vi "Waveform_Generation_SubVI.vi"(8 "ADSR in":dbl[](array[numeric]), 11 "Main Data Cluster in":T1={"Notes Frequency Array"=[], "Main Waveform Type"=enum."Sine", "Waveform"={"t0"=timestamp(0 s since 1904-01-01), "dt"=1.0, "Y"=[]}, "Main Current Note"=0, "Octave Range Offset"=0, "sound format"={"sample rate (S/s)"=22050.0, "number of channels"=2, "bits per sample"=16}, "Task ID"=0, "Note Duration"=0.0, "Volume"=0.0, "ADSR Envelope Cluster"={"Decay"=0, "Sustain"=0, "Attack"=0, "Release"=0}, "Playing?"=FALSE, "Pitch LFO"={"Rate"=0.0, "Ammount"=0.0}, "device ID"=0, "Filter Section"={"Lowpass Freq"=0.0, "Highpass Freq"=0.0, "Enable"=FALSE}, "Distortion"={"Distortion level"=0.0, "Enable"=FALSE}, "Secondary Waveform Type"=enum."Sine", "Secondary Frequency"=0.0, "Secondary Blend"=0.0, "Envelope XY Graph"={[], []}, "Buffer Number"=0, "End of Sequence?"=FALSE} {"task ID" format="%.0x"}) -> (2 "Signal Array out":dbl[](array[numeric]), 3 "dt out":dbl)   [LabVIEW 2019]
doc: "This SubVI generates a specified waveform.\n\nIN: Note Duration in; Sample Rate in; Note Freq in; Waveform Type in; Envelope Array in;\nOUT: dt out; Signal Array out;"
uses:
  <vilib>/Analysis/NI_AALBase.lvlib
  <vilib>/numeric/Random Number (Range) DBL.vi
  controls/#typedef_Waveform_Type.ctl
  <vilib>/sound2/lvsound2.llb/Sound Data Format.ctl
  <vilib>/sound2/lvsound2.llb/Sound Output Task ID.ctl
  controls/#typedef_Data_Cluster.ctl
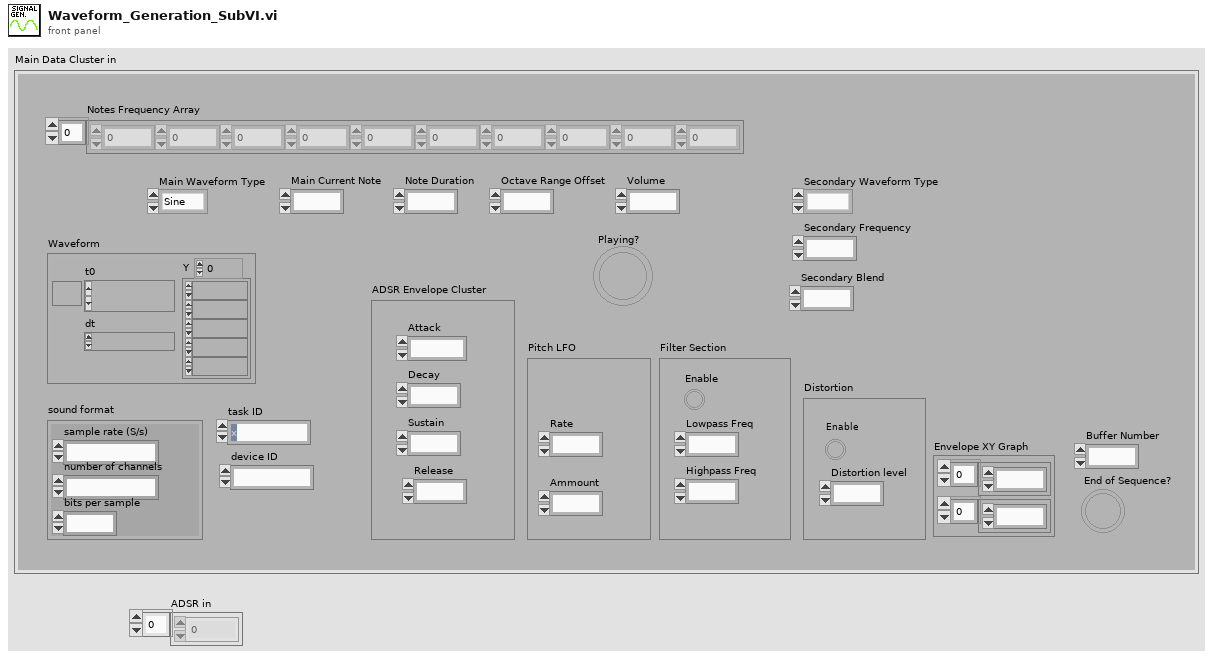
[diagram p1: front panel]
types:
  T1 = typedef "#typedef_Data_Cluster.ctl" = cluster{"Notes Frequency Array":dbl[], "Main Waveform Type":T2, "Waveform":waveform(dbl), "Main Current Note":i32, "Octave Range Offset":u32, "sound format":T3, "Task ID":T4, "Note Duration":dbl, "Volume":dbl, "ADSR Envelope Cluster":cluster{"Decay":i32, "Sustain":i32, "Attack":i32, "Release":i32}, "Playing?":bool, "Pitch LFO":cluster{"Rate":dbl, "Ammount":dbl}, "device ID":u32, "Filter Section":cluster{"Lowpass Freq":dbl, "Highpass Freq":dbl, "Enable":bool}, "Distortion":cluster{"Distortion level":dbl, "Enable":bool}, "Secondary Waveform Type":T2, "Secondary Frequency":dbl, "Secondary Blend":dbl, "Envelope XY Graph":cluster{dbl[], dbl[]}, "Buffer Number":i32, "End of Sequence?":bool}
  T2 = typedef "#typedef_Waveform_Type.ctl" = enum16{"Sine", "Saw", "Square", "Triangle", "Noise"}
  T3 = typedef "Sound Data Format.ctl" = cluster{"sample rate (S/s)":dbl, "number of channels":i32, "bits per sample":i32}
  T4 = typedef "Sound Output Task ID.ctl" = u32
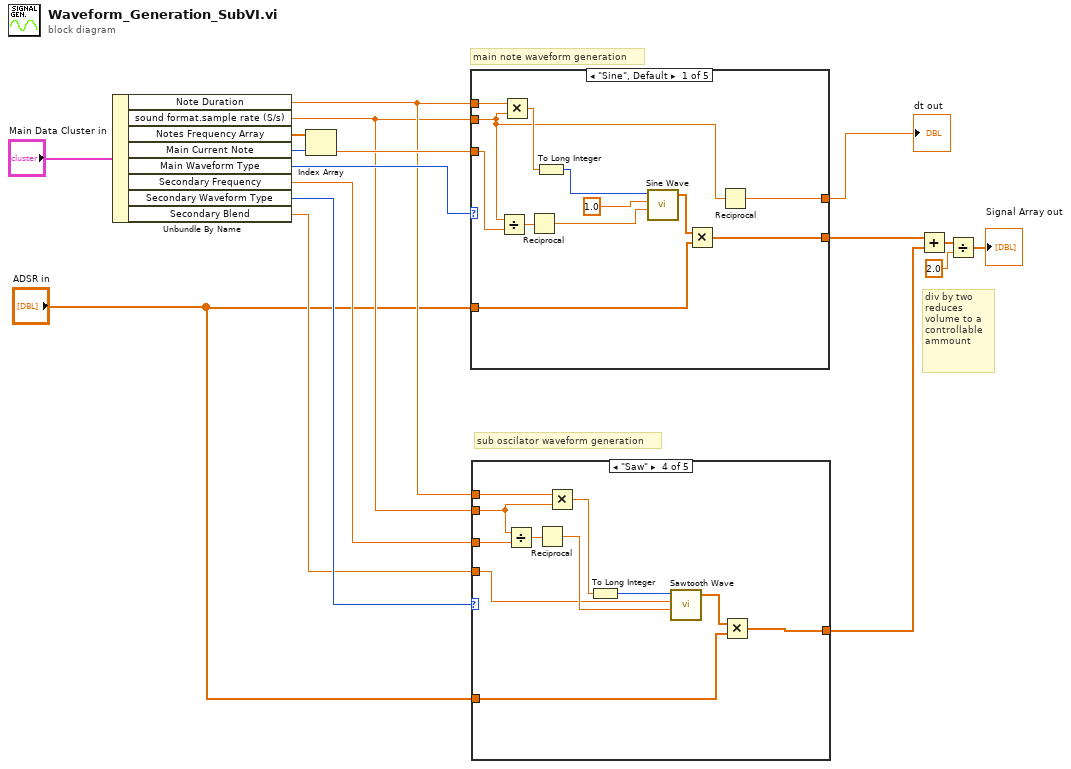
[diagram p0: block diagram]
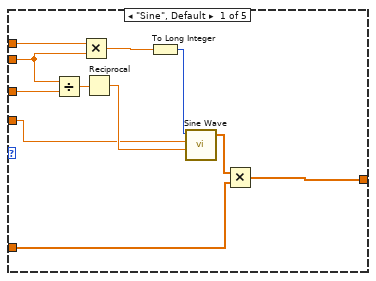
[diagram p2: hidden frame]
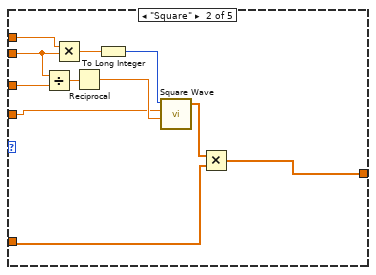
[diagram p3: hidden frame]
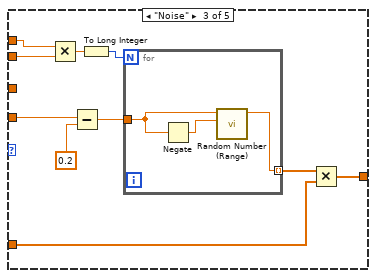
[diagram p4: hidden frame]
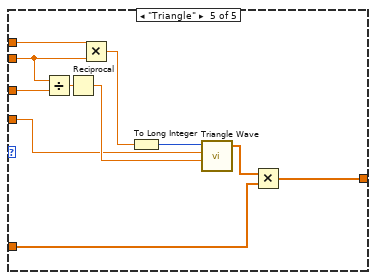
[diagram p5: hidden frame]
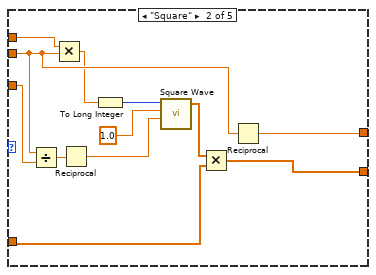
[diagram p6: hidden frame]
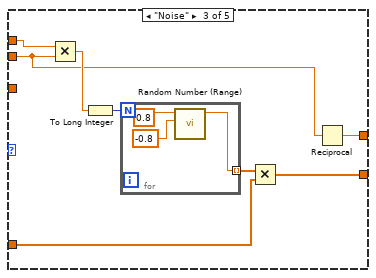
[diagram p7: hidden frame]
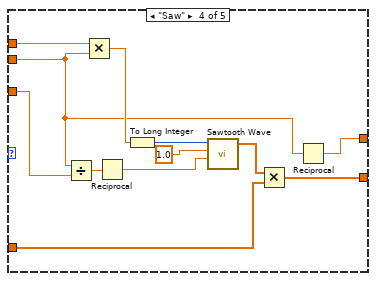
[diagram p8: hidden frame]
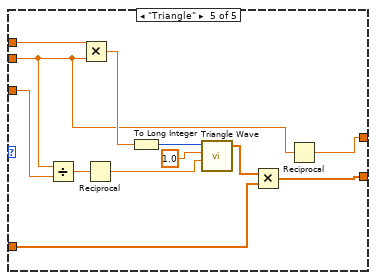
[diagram p9: hidden frame]
diagram:
  # "div by two reduces volume to a controllable ammount"
  # "main note waveform generation"
  # "sub oscilator waveform generation"
  n1 = Unbundle By Name("Main Data Cluster in") -> ("Note Duration"=w11:dbl, "sound format.sample rate (S/s)"=w10:dbl, "Notes Frequency Array"=w15:dbl[], "Main Current Note"=w16:i32, "Main Waveform Type"=w13:T2, "Secondary Frequency"=w9:dbl, "Secondary Waveform Type"=w8:T2, "Secondary Blend"=w7:dbl)
  n2 = Index Array(array=w15, index=w16) -> (element=w14:dbl)
  n3 = case shown="\"Sine\", Default" w13 {
    tunnel: w14 -> [w28 w40 _ w61 w71]
    tunnel: w10 -> [w24 w37 w44 w55 w67]
    tunnel: w11 -> [w27 w39 w48 w62 w74]
    tunnel: "ADSR in" -> [w25 w38 w45 w58 w70]
    tunnel: [w19 w31 w43 w54 w66] -> w17
    tunnel: [w18 w30 w42 w53 w65] -> w3
    frame "Sine", Default {
      n4 = Divide(x=w24, y=w28) -> (x/y=w29:dbl)
      n5 = Multiply(x=w27, y=w24) -> (x*y=w26:dbl)
      n6 = Reciprocal(x=w29) -> (1/x=w20:dbl)
      n7 = To Long Integer(number=w26) -> (32bit integer=w23:i32)
      n8 = call <vilib>:"Sine Wave.vi"("samples"=w23, "amplitude"=1.0, "frequency"=w20) -> ("sine wave"=w21:dbl[])  [unwired: 2 in, 2 out]
      n9 = Multiply(x=w21, y=w25) -> (x*y=w18:dbl[])
      n10 = Reciprocal(x=w24) -> (1/x=w19:dbl)
    }
    frame "Square" {
      n11 = Divide(x=w37, y=w40) -> (x/y=w41:dbl)
      n12 = Multiply(x=w39, y=w37) -> (x*y=w36:dbl)
      n13 = Reciprocal(x=w41) -> (1/x=w32:dbl)
      n14 = To Long Integer(number=w36) -> (32bit integer=w34:i32)
      n15 = call <vilib>:"Square Wave.vi"("samples"=w34, "amplitude"=1.0, "frequency"=w32) -> ("square wave"=w33:dbl[])  [unwired: 3 in, 2 out]
      n16 = Multiply(x=w33, y=w38) -> (x*y=w30:dbl[])
      n17 = Reciprocal(x=w37) -> (1/x=w31:dbl)
    }
    frame "Noise" {
      n18 = Multiply(x=w48, y=w44) -> (x*y=w47:dbl)
      n19 = To Long Integer(number=w47) -> (32bit integer=w49:i32)
      n20 = for {
        N: w49 -> [_]
        tunnel: [w50] -> w46 mode=indexing
        n21 = call-poly <vilib>:"Random Number (Range).vi"("lower bound (0)"=-0.8, "upper bound (100)"=0.8) -> ("number"=w50:dbl)  [unwired: 9 in]
      }
      n22 = Multiply(x=w46, y=w45) -> (x*y=w42:dbl[])
      n23 = Reciprocal(x=w44) -> (1/x=w43:dbl)
    }
    frame "Saw" {
      n24 = Divide(x=w55, y=w61) -> (x/y=w60:dbl)
      n25 = Multiply(x=w62, y=w55) -> (x*y=w56:dbl)
      n26 = Reciprocal(x=w60) -> (1/x=w59:dbl)
      n27 = To Long Integer(number=w56) -> (32bit integer=w63:i32)
      n28 = call <vilib>:"Sawtooth Wave.vi"("samples"=w63, "amplitude"=1.0, "frequency"=w59) -> ("sawtooth wave"=w57:dbl[])  [unwired: 2 in, 2 out]
      n29 = Multiply(x=w57, y=w58) -> (x*y=w53:dbl[])
      n30 = Reciprocal(x=w55) -> (1/x=w54:dbl)
    }
    frame "Triangle" {
      n31 = Divide(x=w67, y=w71) -> (x/y=w72:dbl)
      n32 = Multiply(x=w74, y=w67) -> (x*y=w68:dbl)
      n33 = Reciprocal(x=w72) -> (1/x=w73:dbl)
      n34 = To Long Integer(number=w68) -> (32bit integer=w75:i32)
      n35 = call <vilib>:"Triangle Wave.vi"("samples"=w75, "amplitude"=1.0, "frequency"=w73) -> ("triangle wave"=w69:dbl[])  [unwired: 2 in, 2 out]
      n36 = Multiply(x=w69, y=w70) -> (x*y=w65:dbl[])
      n37 = Reciprocal(x=w67) -> (1/x=w66:dbl)
    }
  }
  "dt out" <- w17
  n38 = case shown="\"Saw\"" w8 {
    tunnel: w9 -> [w86 w97 _ w120 w129]
    tunnel: w10 -> [w82 w94 w103 w114 w125]
    tunnel: w11 -> [w85 w96 w107 w121 w132]
    tunnel: "ADSR in" -> [w83 w95 w104 w117 w128]
    tunnel: [w78 w89 w102 w113 w124] -> w4
    tunnel: w7 -> [w77 w88 w101 w112 w123]
    frame "Sine", Default {
      n39 = Divide(x=w82, y=w86) -> (x/y=w87:dbl)
      n40 = Multiply(x=w85, y=w82) -> (x*y=w84:dbl)
      n41 = Reciprocal(x=w87) -> (1/x=w79:dbl)
      n42 = To Long Integer(number=w84) -> (32bit integer=w81:i32)
      n43 = call <vilib>:"Sine Wave.vi"("samples"=w81, "amplitude"=w77, "frequency"=w79) -> ("sine wave"=w80:dbl[])  [unwired: 2 in, 2 out]
      n44 = Multiply(x=w80, y=w83) -> (x*y=w78:dbl[])
    }
    frame "Square" {
      n45 = Divide(x=w94, y=w97) -> (x/y=w98:dbl)
      n46 = Multiply(x=w96, y=w94) -> (x*y=w93:dbl)
      n47 = Reciprocal(x=w98) -> (1/x=w90:dbl)
      n48 = To Long Integer(number=w93) -> (32bit integer=w92:i32)
      n49 = call <vilib>:"Square Wave.vi"("samples"=w92, "amplitude"=w88, "frequency"=w90) -> ("square wave"=w91:dbl[])  [unwired: 3 in, 2 out]
      n50 = Multiply(x=w91, y=w95) -> (x*y=w89:dbl[])
    }
    frame "Noise" {
      n51 = Multiply(x=w107, y=w103) -> (x*y=w106:dbl)
      n52 = Subtract(x=w101, y=0.2) -> (x-y=w99:dbl)
      n53 = To Long Integer(number=w106) -> (32bit integer=w108:i32)
      n54 = for {
        N: w108 -> [_]
        tunnel: [w111] -> w105 mode=indexing
        tunnel: w99 -> [w109]
        n55 = Negate(x=w109) -> (-x=w110:dbl)
        n56 = call-poly <vilib>:"Random Number (Range).vi"("lower bound (0)"=w110, "upper bound (100)"=w109) -> ("number"=w111:dbl)  [unwired: 9 in]
      }
      n57 = Multiply(x=w105, y=w104) -> (x*y=w102:dbl[])
    }
    frame "Saw" {
      n58 = Divide(x=w114, y=w120) -> (x/y=w119:dbl)
      n59 = Reciprocal(x=w119) -> (1/x=w118:dbl)
      n60 = Multiply(x=w121, y=w114) -> (x*y=w115:dbl)
      n61 = To Long Integer(number=w115) -> (32bit integer=w122:i32)
      n62 = call <vilib>:"Sawtooth Wave.vi"("samples"=w122, "amplitude"=w112, "frequency"=w118) -> ("sawtooth wave"=w116:dbl[])  [unwired: 2 in, 2 out]
      n63 = Multiply(x=w116, y=w117) -> (x*y=w113:dbl[])
    }
    frame "Triangle" {
      n64 = Divide(x=w125, y=w129) -> (x/y=w130:dbl)
      n65 = Reciprocal(x=w130) -> (1/x=w131:dbl)
      n66 = Multiply(x=w132, y=w125) -> (x*y=w126:dbl)
      n67 = To Long Integer(number=w126) -> (32bit integer=w133:i32)
      n68 = call <vilib>:"Triangle Wave.vi"("samples"=w133, "amplitude"=w123, "frequency"=w131) -> ("triangle wave"=w127:dbl[])  [unwired: 2 in, 2 out]
      n69 = Multiply(x=w127, y=w128) -> (x*y=w124:dbl[])
    }
  }
  n70 = Add(x=w3, y=w4) -> (x+y=w6:dbl[])
  n71 = Divide(x=w6, y=2.0) -> (x/y=→"Signal Array out":dbl[])
